vi "vollath_calculation_focus_algorithm_serge_doug.vi"(1 "Array":dbl[][](array[numeric])) -> (0 "VollVal":dbl)   [LabVIEW 2011]
doc: "Calculates a goodness-of-focus parameter using the Vollath autocorrelation algorithm (Vollath, D. (1987). Automatic focusing by correlative methods. J. Microsc. 147 pp 279-288.) See Santos, A., Ortiz de Solorzano, C., Vaquero, J. J., Pena, J. M., Malpica, N., and del Pozo, F. (1997). Evaluation of autofocus functions in molecular cytogenetic analysis. J Microsc 188 (Pt 3), 264-272 for a more general discussion of autofocusing algorithms in light microscopy."
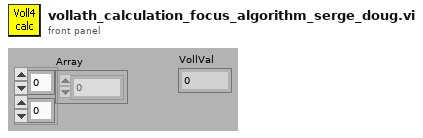
[diagram p1: front panel]
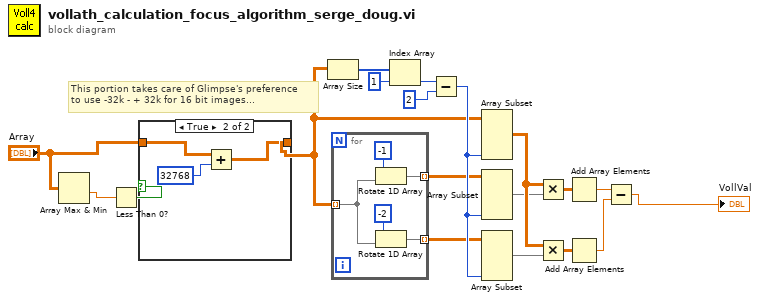
[diagram p0: block diagram]
diagram:
  # "This portion takes care of Glimpse's preference\nto use -32k - + 32k for 16 bit images..."
  n1 = Array Max & Min(array="Array") -> (min value=w2:dbl)  [unwired: 3 out]
  n2 = Less Than 0?(x=w2) -> (x < 0?=w1:bool)
  n3 = case shown="True" w1 {
    tunnel: "Array" -> [w20 w23]
    tunnel: [w20 w22] -> w3
    frame False {
      # "The min is bigger\nthan zero - leave\nalone"
    }
    frame True {
      n4 = Add(x=w23, y=32768) -> (x+y=w22:dbl[][])
    }
  }
  n5 = Array Size(array=w3) -> (size(s)=w18:i32[])
  n6 = for {
    tunnel: w3 -> [w26] mode=indexing
    tunnel: [w25] -> w6 mode=indexing
    tunnel: [w24] -> w7 mode=indexing
    n7 = Rotate 1D Array(1:w26, 2:-1 ("n")) -> (0:w25:dbl[])
    n8 = Rotate 1D Array(1:w26, 2:-2 ("n")) -> (0:w24:dbl[])
  }
  n9 = Index Array(array=w18, index=1) -> (element=w9:i32)
  n10 = Subtract(x=w9, y=2) -> (x-y=w19:i32)
  n11 = Array Subset(array=w3, length (col)=w19) -> (w12:dbl[][])  [unwired: 3 in]
  n12 = Array Subset(array=w6, length (col)=w19) -> (w11:dbl[][])  [unwired: 3 in]
  n13 = Array Subset(array=w7, length (col)=w19) -> (w13:dbl[][])  [unwired: 3 in]
  n14 = Multiply(x=w12, y=w11) -> (x*y=w14:dbl[][])
  n15 = Multiply(x=w12, y=w13) -> (x*y=w15:dbl[][])
  n16 = Add Array Elements(numeric array=w14) -> (sum=w16:dbl)
  n17 = Add Array Elements(numeric array=w15) -> (sum=w17:dbl)
  n18 = Subtract(x=w16, y=w17) -> (x-y=→"VollVal":dbl)
